vi "Init.vi"(8 "error in (no error)":errorcluster, 9 "SA Pin":string, 10 "Measurement Name":string) -> (0 "error out":errorcluster, 3 "GSM_PVT_out":refnum<class "GSM_PVT.lvclass">)   [LabVIEW 2016, in "SeqAuto Evaluations.lvlib" / "GSM_PVT.lvclass"]
uses:
  GSM_PVT.lvclass
  C:/Sequence Automation/Plugins/SeqAuto IEvaluation.lvlibp/SeqAuto IEvaluation.lvclass
  GSM_PVT.lvclass/GSM_PVT.ctl
  Plugins/SeqAuto IEvaluation.lvlibp/Write Measurement Name.vi
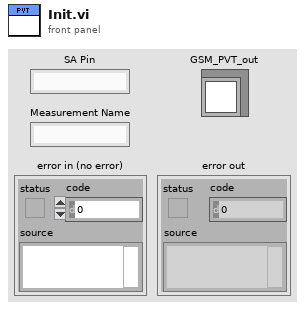
[diagram p1: front panel]
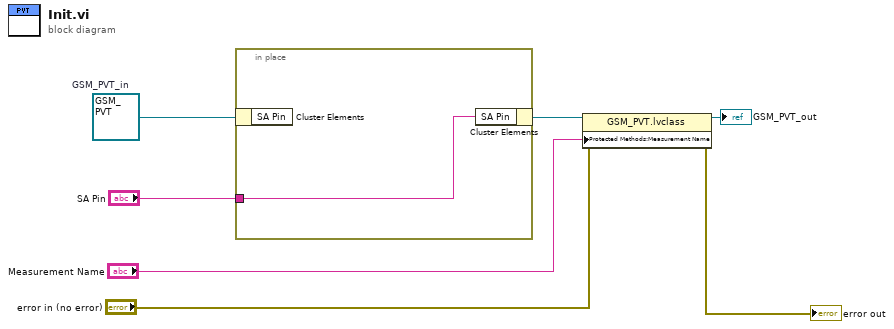
[diagram p0: block diagram]
diagram:
  w2 = refnum<class "GSM_PVT.lvclass"> refnum  # GSM_PVT_in
  n1 = in-place {
    in-place-border: "SA Pin" -> [w8]
    n2 = in-place-cluster #1(w2) -> ()  [unwired: 1 out]
    n3 = in-place-cluster #1("SA Pin"=w8) -> (w4:refnum<class "GSM_PVT.lvclass">)
  }
  n4 = property class="GSM_PVT.lvclass"(reference=w4, error in="error in (no error)", "Protected Methods:Measurement Name"="Measurement Name") -> (reference out=→"GSM_PVT_out":refnum<class "GSM_PVT.lvclass">, error out=→"error out":errorcluster)
